vi "AppConfigJSON_Create.vi"(8 "ErrorIn":errorcluster, 11 "ReferenceIn":refnum<class "AppConfigJSON.lvclass">) -> (0 "ErrorOut":errorcluster, 3 "ReferenceOut":refnum<class "AppConfigJSON.lvclass">)   [LabVIEW 2021, in "AppConfigJSON.lvclass"]
uses:
  AppConfigJSON.lvclass
  AppConfigJSON.lvclass/AppConfigJSON.ctl
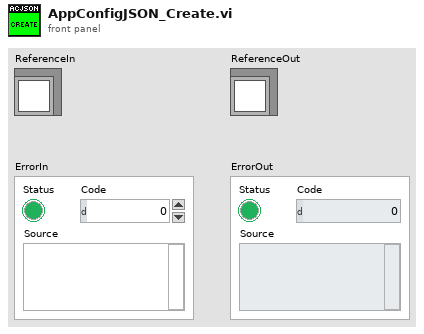
[diagram p1: front panel]
types:
  T1 = typedef "AppConfigJSON.lvclass/ObjectAttributes.ctl" = cluster{"Name":string, "ConfigFilePath":path, "Objects":T2[], "ApplicationBasePath":path, "ObjectName":string}
  T2 = typedef "IApplicationConfiguration.lvclass/ObjectDataDetails.ctl" = cluster{"ObjectName":string, "ObjectType":string, "Interfaces":T3[]}
  T3 = typedef "IApplicationConfiguration.lvclass/ObjectData.ctl" = cluster{"Label":string, "ObjectName":string, "Type":string}
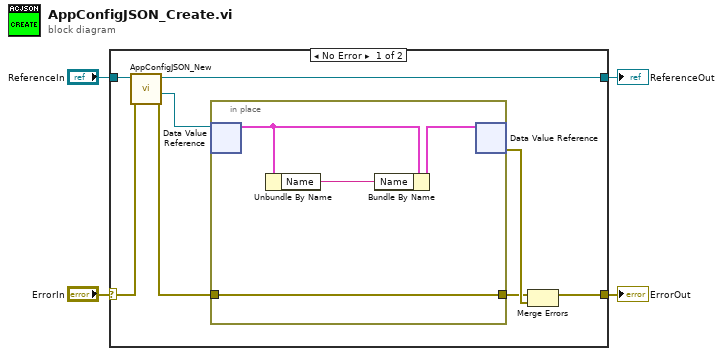
[diagram p0: block diagram]
diagram:
  n1 = case shown="No Error" "ErrorIn" {
    selector: "ErrorIn" -> [w12 w18]
    tunnel: [w8 w18] -> w3
    tunnel: "ReferenceIn" -> [w7 w17]
    tunnel: [w6 w17] -> w1
    frame No Error {
      n2 = call "AppConfigJSON_New.vi"("ErrorIn"=w12, "ReferenceIn"=w7) -> ("ErrorOut"=w10:errorcluster, "DVRRefOut"=w5:refnum<data-value>, "ReferenceOut"=w6:refnum<class "AppConfigJSON.lvclass">)  [unwired: 6 in, 1 out]
      n3 = in-place {
        in-place-border: w10 -> [w16]
        in-place-border: [w16] -> w9
        n4 = in-place-dvr #1(w5) -> (w14:T1)  [unwired: 1 out]
        n5 = Unbundle By Name(w14) -> ("Name"=w13:string)
        n6 = Bundle By Name(cluster=w14, "Name"=w13) -> (w15:T1)
        n7 = in-place-dvr #1(w15) -> (w11:errorcluster)  [unwired: 1 out]
      }
      n8 = Merge Errors(w9, w11) -> (w8:errorcluster)
    }
    frame Error {
      # "VI-TechBaseTemplate_Simple_4x4x4"
    }
  }
  "ErrorOut" <- w3
  "ReferenceOut" <- w1
